vi "ARM_BEGIN.vi"(8 "error in":errorcluster) -> (0 "error out":errorcluster)   [LabVIEW 2023]
uses:
  <vilib>/Rock Robotics/WPI/ThirdParty/Phoenix-LabVIEW/Motor Controller/Controls/CTRE_Phoenix_MotorControl_TalonFXInvertType.ctl
  <vilib>/Rock Robotics/WPI/ThirdParty/Phoenix-LabVIEW/Motor Controller/Controls/CTRE_Phoenix_MotorControl_FeedbackDevice_TalonFX.ctl
  <vilib>/Rock Robotics/WPI/ThirdParty/Phoenix-LabVIEW/Motor Controller/Controls/CTRE_Phoenix_MotorControl_NeutralMode.ctl
  <vilib>/Rock Robotics/WPI/ThirdParty/Phoenix-LabVIEW/CANCoder/Controls/CTRE_Phoenix_CANcoder_StatusFrame.ctl
  <vilib>/Rock Robotics/WPI/ThirdParty/Phoenix-LabVIEW/CANCoder/Controls/CTRE_Phoenix_CANcoder_SensorInitializationStrategy.ctl
  <vilib>/Rock Robotics/WPI/ThirdParty/JAS_Junk/TrajLib/Enum/DCMOTOR_TYPES_ENUM.ctl
  ARM_GLOBALS.vi
  <vilib>/Rock Robotics/WPI/ThirdParty/JAS_Junk/TrajLib/Trajectory_Library.lvlib
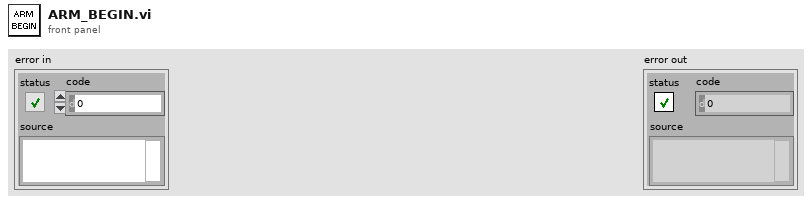
[diagram p1: front panel]
types:
  T1 = typedef "Trajectory_Library.lvlib/DCMOTOR_TYPES_ENUM.ctl" = enum16{"CIM", "AndyMark 9015", "Andy Mark RS 775 125", "Bag", "BaneBots RS 550", "BaneBots RS 775", "Falcon 500", "Mini CIM", "NEO", "NEO 550", "Romi BuiltIn", "Vex 775 Pro", "Snow Blower AM 2235A", "Bosch Seat AM 3493"}
  T2 = typedef "CTRE_Phoenix_CANcoder_SensorInitializationStrategy.ctl" = enum16{"Boot To Zero", "Boot To Absolute Position"}
  T3 = typedef "CTRE_Phoenix_CANcoder_StatusFrame.ctl" = u32
  T4 = typedef "CTRE_Phoenix_MotorControl_NeutralMode.ctl" = enum8{"EEPROMSetting", "Override to Coast", "Override to Brake"}
  T5 = typedef "CTRE_Phoenix_MotorControl_FeedbackDevice_TalonFX.ctl" = i8
  T6 = typedef "CTRE_Phoenix_MotorControl_TalonFXInvertType.ctl" = enum16{"Counter-Clockwise", "Clockwise"}
  T7 = typedef "WPI_MotorControlDeviceRef.ctl" = cluster{"DeviceStatus":errorcluster, "Type":T8, "PWM":cluster{"PWM Channel":T9, "DeadBand":T10}, "CAN":cluster{"Device Number":u8, "SetOutput VI Ref":variant, "GetOutput VI Ref":variant, "Enable VI Ref":variant, "Disable VI Ref":variant, "Data":variant}, "Invert":bool, "DIO PWM":cluster{"PWM \"Enable\" Channel":T9, "DIOChannel":T11, "PWM Rate":dbl}}
  T8 = typedef "WPI_MotorControlType.ctl" = enum16{"PWM", "CAN", "DIO PWM"}
  T9 = typedef "FPGA_DIOPWMChannel.ctl" = enum8{"PWM 0", "PWM 1", "PWM 2", "PWM 3", "PWM 4", "PWM 5", "PWM 6", "PWM 7", "PWM 8", "PWM 9", "PWM MXP 0", "PWM MXP 1", "PWM MXP 2", "PWM MXP 3", "PWM MXP 4", "PWM MXP 5", "PWM MXP 6", "PWM MXP 7", "PWM MXP 8", "PWM MXP 9", "Invalid"}
  T10 = typedef "WPI_PWMDeadband.ctl" = cluster{"Name":string, "maxPositivePwm":i32, "minPositivePwm":i32, "centerPwm":i32, "maxNegativePwm":i32, "minNegativePwm":i32, "angularRange":u16}
  T11 = typedef "FPGA_DIOChannel.ctl" = enum8{"DIO 0", "DIO 1", "DIO 2", "DIO 3", "DIO 4", "DIO 5", "DIO 6", "DIO 7", "DIO 8", "DIO 9", "DIO MXP 0", "DIO MXP 1", "DIO MXP 2", "DIO MXP 3", "DIO MXP 4", "DIO MXP 5", "DIO MXP 6", "DIO MXP 7", "DIO MXP 8", "DIO MXP 9", "DIO MXP 10", "DIO MXP 11", "DIO MXP 12", "DIO MXP 13", "DIO MXP 14", "DIO MXP 15", "SPI Port CS1", "SPI Port CS2", "SPI Port CS3", "SPI Port MISO", "SPI Port MOSI", "Invalid"}
  T12 = typedef "CTRE_Phoenix_CANcoder_DeviceRef.ctl" = cluster{"DeviceStatus":errorcluster, "Device Number":u8, "Handle":u64, "UsageFrame":u32, "Library Path":path}
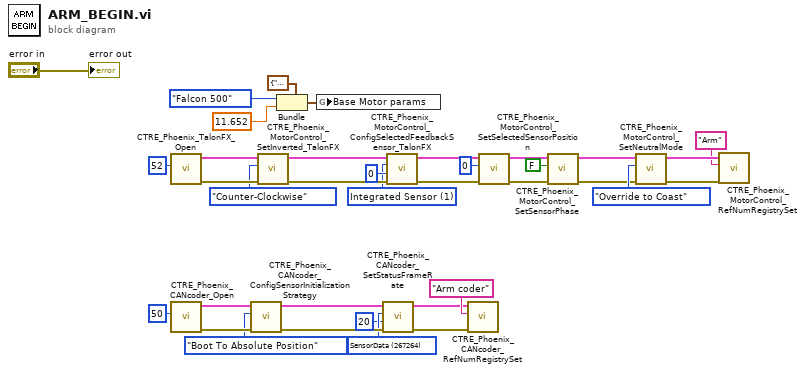
[diagram p0: block diagram]
diagram:
  w26 = T3 267264 items=["SensorData"=267264, "VbatAndFaults"=267328] ("CANcoder Status Frame")
  w13 = T5 1 items=["Integrated Sensor"=1, "Sensor Sum (S0 + S1)"=9, "Sensor Difference (D0 - D1)"=10, "Remote Source 0"=11, "Remote Source 1"=12, "None"=14, "Software Emulated"=15] ("Talon FX Feedback Device")
  n1 = call <vilib>:"CTRE_Phoenix_TalonFX_Open.vi"("Device Number"=u8 52) -> ("error out"=w19:errorcluster, "PhoenixMotorControlDevRef"=w18:T7)  [unwired: 9 in]
  n2 = call <vilib>:"CTRE_Phoenix_CANcoder_Open.vi"("Device Number"=50) -> ("error out"=w32:errorcluster, "CTRE_CANcoder_DeviceRef"=w30:T12)  [unwired: 9 in]
  n3 = call <vilib>:"CTRE_Phoenix_CANcoder_ConfigSensorInitializationStrategy.vi"("error in"=w32, "Sensor Initialization Strategy"=CTRE_Phoenix_CANcoder_SensorInitializationStrategy."Boot To Absolute Position", "CTRE_CANcoder_DeviceRef"=w30) -> ("error out"=w33:errorcluster, "CTRE_CANcoder_DeviceRef"=w31:T12)  [unwired: 7 in]
  n4 = call <vilib>:"CTRE_Phoenix_MotorControl_SetInverted_TalonFX.vi"("error in (no error)"=w19, "Invert Type"=CTRE_Phoenix_MotorControl_TalonFXInvertType."Counter-Clockwise", "PhoenixMotorControlDevRef"=w18) -> ("error out"=w15:errorcluster, "PhoenixMotorControlDevRef"=w14:T7)  [unwired: 7 in]
  n5 = Bundle(cluster=cluster{"Motor Type":T1, "Gear Ratio":dbl} {"Motor Type"=enum."CIM", "Gear Ratio"=0.0} ("Base Motor params"), "Motor Type"=DCMOTOR_TYPES_ENUM."Falcon 500", "Gear Ratio"=11.652) -> (w3:cluster{"Motor Type":T1, "Gear Ratio":dbl})
  n6 = global write "ARM_GLOBALS.vi" "Base Motor params"(w3) -> ()
  n7 = call <vilib>:"CTRE_Phoenix_CANcoder_SetStatusFrameRate.vi"("error in (no error)"=w33, "Period (ms)"=u8 20, "CANcoder Status Frame"=w26, "CTRE_CANcoder_DeviceRef"=w31) -> ("error out"=w23:errorcluster, "CTRE_CANcoder_DeviceRef"=w24:T12)  [unwired: 6 in]
  n8 = call <vilib>:"CTRE_Phoenix_MotorControl_ConfigSelectedFeedbackSensor_TalonFX.vi"("error in (no error)"=w15, "pidLoopIdx"=0, "Talon FX Feedback Device"=w13, "PhoenixMotorControlDevRef"=w14) -> ("error out"=w8:errorcluster, "PhoenixMotorControlDevRef"=w9:T7)  [unwired: 6 in]
  n9 = call <vilib>:"CTRE_Phoenix_CANcoder_RefNumRegistrySet.vi"("error in (no error)"=w23, "refnum name"="Arm coder", "CTRE_CANcoder_DeviceRef"=w24) -> ()  [unwired: 7 in, 2 out]
  n10 = call <vilib>:"CTRE_Phoenix_MotorControl_SetSelectedSensorPosition.vi"("error in (no error)"=w8, "New Sensor Position"=0, "PhoenixMotorControlDevRef"=w9) -> ("error out"=w35:errorcluster, "PhoenixMotorControlDevRef"=w34:T7)  [unwired: 7 in]
  n11 = call <vilib>:"CTRE_Phoenix_MotorControl_SetSensorPhase.vi"("error in (no error)"=w35, "PhaseSensor"=FALSE, "PhoenixMotorControlDevRef"=w34) -> ("error out"=w6:errorcluster, "PhoenixMotorControlDevRef"=w7:T7)  [unwired: 7 in]
  n12 = call <vilib>:"CTRE_Phoenix_MotorControl_SetNeutralMode.vi"("error in (no error)"=w6, "Motor Control Neutral Mode"=CTRE_Phoenix_MotorControl_NeutralMode."Override to Coast", "PhoenixMotorControlDevRef"=w7) -> ("error out"=w22:errorcluster, "PhoenixMotorControlDevRef"=w21:T7)  [unwired: 7 in]
  n13 = call <vilib>:"CTRE_Phoenix_MotorControl_RefNumRegistrySet.vi"("error in (no error)"=w22, "refnum name"="Arm", "PhoenixMotorControlDevRef"=w21) -> ()  [unwired: 7 in, 2 out]
  "error out" <- "error in"
